vi "FGV_cmdQ.vi"(7 "prio":bool, 8 "error in (no error)":errorcluster, 9 "dataIn":variant, 10 "actionIn":string, 11 "Qaction":T1=enum."enqueue") -> (0 "error out":errorcluster, 3 "queue out":refnum<queue>)   [LabVIEW 2014]
uses:
  typeDefs/cmdQaction.ctl
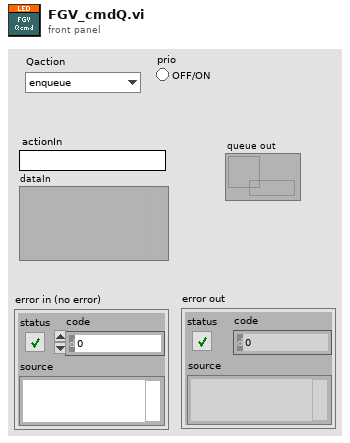
[diagram p1: front panel]
types:
  T1 = typedef "cmdQaction.ctl" = enum16{"create", "enqueue", "getQueue"}
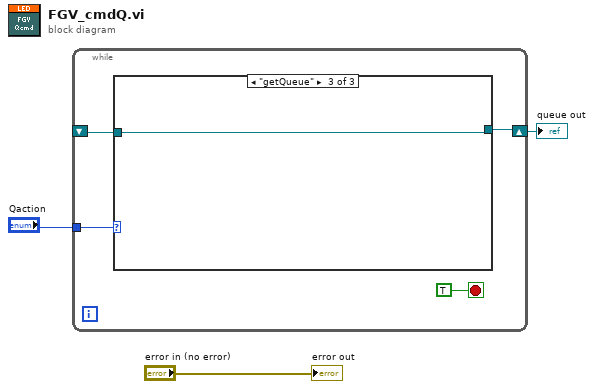
[diagram p0: block diagram]
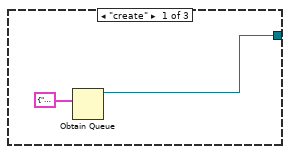
[diagram p2: hidden frame]
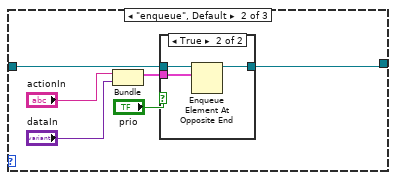
[diagram p3: hidden frame]
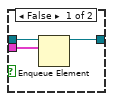
[diagram p4: hidden frame]
diagram:
  n1 = while {
    tunnel: "Qaction" -> [w6]
    shift-right: [w5] -> w1
    shift-left: _ -> [w4]
    stop <- TRUE stop-if-true
    n2 = case shown="\"getQueue\"" w6 {
      tunnel: [w8 w14 w22] -> w5
      tunnel: w4 -> [_ w15 w22]
      frame "create" {
        n3 = Obtain Queue(element data type=cluster{"action":string, "data":variant} {"action"="", "data"=variant} ("Qcmd")) -> (queue out=w8:refnum<queue>)  [unwired: 4 in, 2 out]
      }
      frame "enqueue", Default {
        n4 = Bundle("actionIn"="actionIn", "dataIn"="dataIn") -> (w12:cluster{"actionIn":string, "dataIn":variant})  [unwired: 1 in]
        n5 = case shown="True" "prio" {
          tunnel: w15 -> [w18 w21]
          tunnel: [w17 w19] -> w14
          tunnel: w12 -> [w16 w20]
          frame False {
            n6 = Enqueue Element(queue=w18, element=w16) -> (queue out=w17:refnum<queue>)  [unwired: 2 in, 2 out]
          }
          frame True {
            n7 = Enqueue Element At Opposite End(queue=w21, element=w20) -> (queue out=w19:refnum<queue>)  [unwired: 2 in, 2 out]
          }
        }
      }
      frame "getQueue" {
      }
    }
  }
  "queue out" <- w1
  "error out" <- "error in (no error)"
